vi "load mode fg.vi"(1 "Load Mode":enum16{"Feild Load", "Human Player Load"}(ring), 2 "Menu":T1) -> (0 "Load Mode":enum16{"Feild Load", "Human Player Load"}(ring))   [LabVIEW 2013]
uses:
  typedefs/fg_typedef.ctl
panel:
  # "Load Mode"
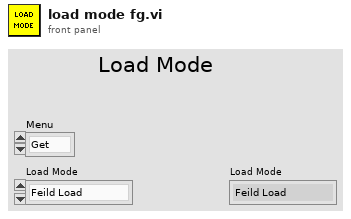
[diagram p1: front panel]
types:
  T1 = typedef "fg_typedef.ctl" = enum16{"Get", "Set"}
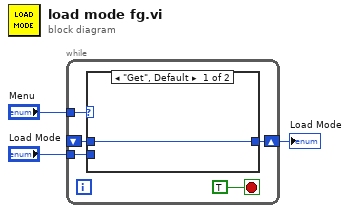
[diagram p0: block diagram]
diagram:
  n1 = while {
    tunnel: "Menu" -> [w7]
    shift-right: [w5] -> w1
    shift-left: _ -> [w4]
    tunnel: "Load Mode" -> [w6]
    stop <- TRUE stop-if-true
    n2 = case shown="\"Get\", Default" w7 {
      tunnel: w6 -> [_ w10]
      tunnel: [w9 w10] -> w5
      tunnel: w4 -> [w9 _]
      frame "Get", Default {
      }
      frame "Set" {
      }
    }
  }
  "Load Mode" <- w1
